vi "7-19-19 data.vi"() -> ()   [LabVIEW 2016]
uses:
  <userlib>/Levylab/LV to ITX/LVtoITX.lvclass
  <vilib>/Analysis/NI_AALPro.lvlib
panel:
  out "dG/dt Vs Temp":cluster{"Data":dbl[], "Data":dbl[]}[](graph)
  out "output cluster":cluster{dbl[], dbl[], dbl[], dbl[]}
  out "G2T Vs Temp":cluster{"Data":dbl[], "Data":dbl[]}[](graph)
  out "Data":dbl[][](array[numeric])
  out "G Vs Time":cluster{"Data":dbl[], "Data":dbl[]}[](graph)
  out "Wavenames":string[](array[string])
  in  "Path":path
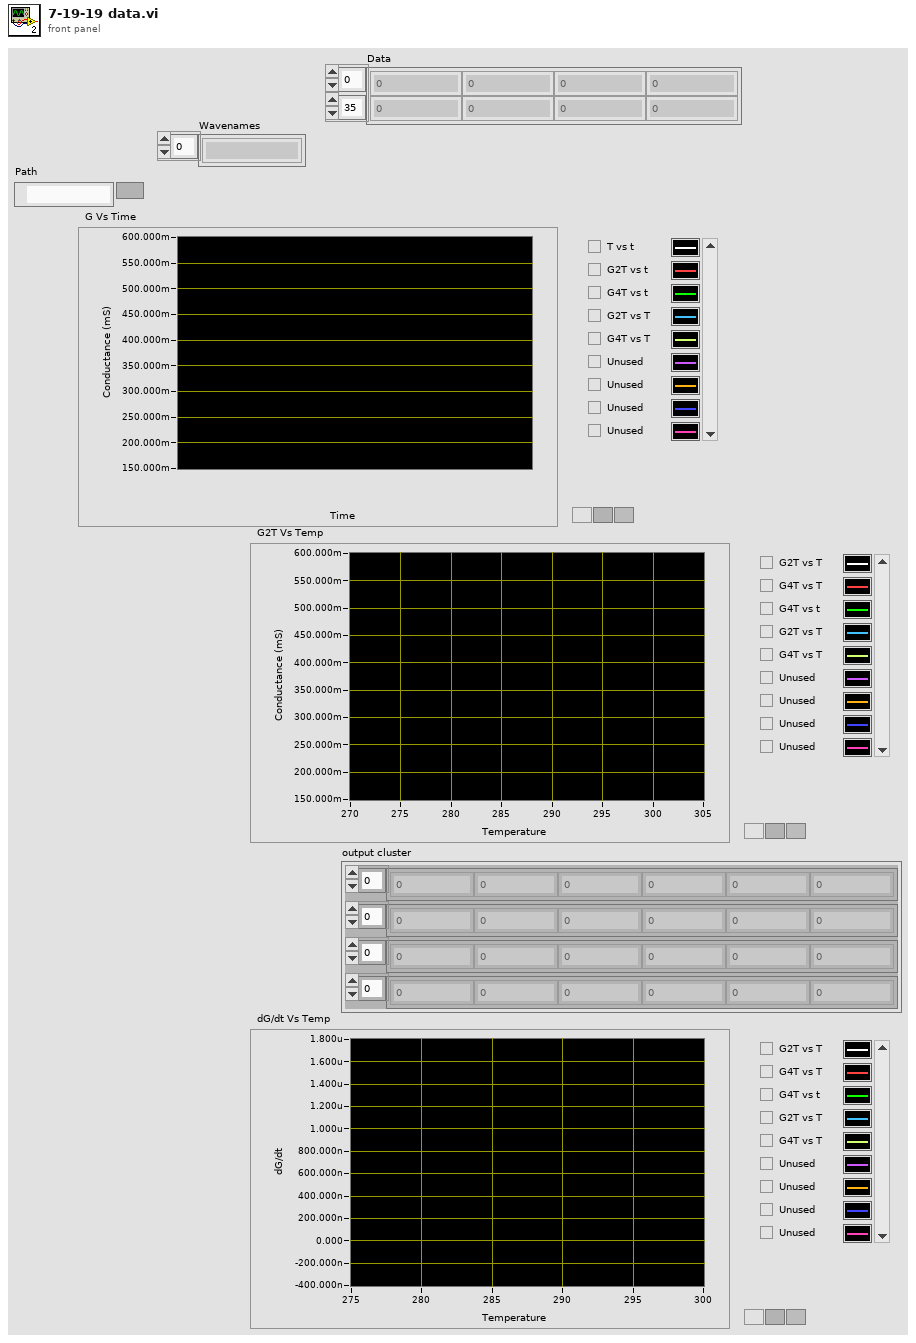
[diagram p1: front panel]
types:
  T1 = cluster{"slope min":dbl, "slope max":dbl, "intercept min":dbl, "intercept max":dbl}
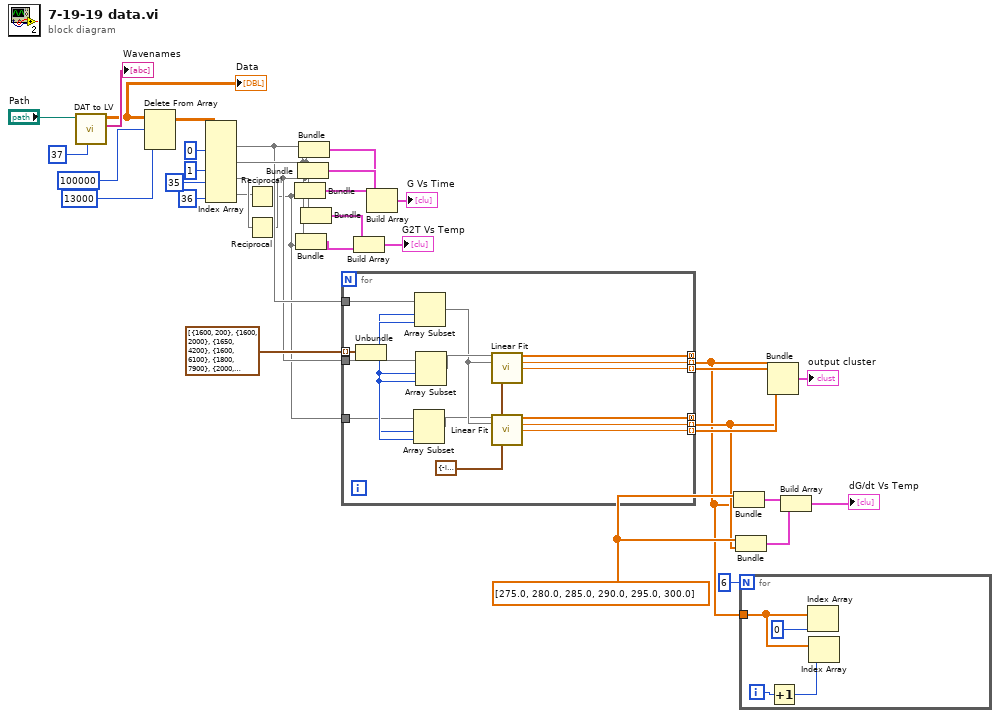
[diagram p0: block diagram]
diagram:
  w8 = dbl[] [275.0, 280.0, 285.0, 290.0, 295.0, 300.0]
  n1 = call <userlib>:"DAT to LV.vi"("header length"=37, "File Path"="Path") -> ("Wavenames"=→"Wavenames":string[], "Data"=w16:dbl[][])  [unwired: 6 in, 2 out]
  "Data" <- w16
  n2 = Delete From Array(array=w16, length=100000, index (row)=13000 ("index")) -> (array with subset deleted=w15:dbl[][])  [unwired: 1 in, 1 out]
  n3 = Index Array(array=w15, index (col) #1=0 ("disabled index (col)"), index (col) #2=1 ("index (col)"), index (col) #3=35 ("index (col)"), index (col) #4=36 ("index (col)")) -> (element #1=w13:dbl[], element #2=w28:dbl[], element #3=w23:dbl[], element #4=w22:dbl[])  [unwired: 4 in]
  n4 = Reciprocal(x=w22) -> (1/x=w11:dbl[])
  n5 = Reciprocal(x=w23) -> (1/x=w12:dbl[])
  n6 = Bundle("Data"=w13, w11) -> (w27:cluster{"Data":dbl[], dbl[]})  [unwired: 1 in]
  n7 = Bundle("Data"=w28, w11) -> (w20:cluster{"Data":dbl[], dbl[]})  [unwired: 1 in]
  n8 = Bundle("Data"=w13, w12) -> (w26:cluster{"Data":dbl[], dbl[]})  [unwired: 1 in]
  n9 = Bundle("Data"=w13, "Data"=w28) -> (w25:cluster{"Data":dbl[], "Data":dbl[]})  [unwired: 1 in]
  n10 = Bundle("Data"=w28, w12) -> (w21:cluster{"Data":dbl[], dbl[]})  [unwired: 1 in]
  n11 = for {
    tunnel: cluster{"length":i32, "index":i32}[] [{"length"=1600, "index"=200}, {"length"=1600, "index"=2000}, {"length"=1650, "index"=4200}, {"length"=1600, "index"=6100}, {"length"=1800, "index"=7900}, {"length"=2000, "index"=10000}] -> [w51] mode=indexing
    tunnel: w13 -> [w48]
    tunnel: w12 -> [w47]
    tunnel: w11 -> [w46]
    tunnel: [w41] -> _ mode=concatenating
    tunnel: [w40] -> _ mode=concatenating
    tunnel: [w39] -> w3 mode=indexing
    tunnel: [w38] -> w10 mode=indexing
    tunnel: [w37] -> w2 mode=indexing
    tunnel: [w36] -> w7 mode=indexing
    w42 = T1 {"slope min"=-inf, "slope max"=inf, "intercept min"=-inf, "intercept max"=inf} ("parameter bounds")
    n12 = Unbundle(w51) -> ("length"=w50:i32, "index"=w49:i32)
    n13 = Array Subset(array=w46, index=w49, length=w50) -> (w43:dbl[])
    n14 = Array Subset(array=w48, index=w49, length=w50) -> (w44:dbl[])
    n15 = Array Subset(array=w47, index=w49, length=w50) -> (w45:dbl[])
    n16 = call <vilib>:"Linear Fit.vi"("Y"=w45, "X"=w44, "parameter bounds"=w42) -> ("Best Linear Fit"=w41:dbl[], "slope"=w37:dbl, "intercept"=w36:dbl)  [unwired: 8 in, 2 out]
    n17 = call <vilib>:"Linear Fit.vi"("Y"=w43, "X"=w44, "parameter bounds"=w42) -> ("Best Linear Fit"=w40:dbl[], "slope"=w39:dbl, "intercept"=w38:dbl)  [unwired: 8 in, 2 out]
  }
  n18 = Build Array(w21, w20) -> (→"G2T Vs Temp":cluster{"Data":dbl[], dbl[]}[])
  n19 = Build Array(w25, w26, w27) -> (→"G Vs Time":cluster{"Data":dbl[], "Data":dbl[]}[])
  n20 = Bundle(w8, w2) -> (w5:cluster{dbl[], dbl[]})  [unwired: 1 in]
  n21 = Bundle(w8, w3) -> (w6:cluster{dbl[], dbl[]})  [unwired: 1 in]
  n22 = for {
    N: 6 -> [_]
    tunnel: w2 -> [w55]
    i -> [w53]
    n23 = Increment(x=w53) -> (x+1=w52:i32)
    n24 = Index Array(array=w55, index=0) -> ()  [unwired: 1 out]
    n25 = Index Array(array=w55, index=w52) -> ()  [unwired: 1 out]
  }
  n26 = Bundle(w2, w7, w3, w10) -> (→"output cluster":cluster{dbl[], dbl[], dbl[], dbl[]})  [unwired: 1 in]
  n27 = Build Array(w5, w6) -> (→"dG/dt Vs Temp":cluster{dbl[], dbl[]}[])
